vi "数据保存表格-1.vi"(1 "路径":path=path "F:/data", 2 "时间格式字符串(%c)":string="%y年%m月%d日%H 时%M 分%S秒") -> (0 "添加的路径":path)   [LabVIEW 2018]
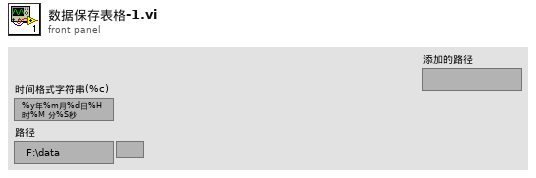
[diagram p1: front panel]
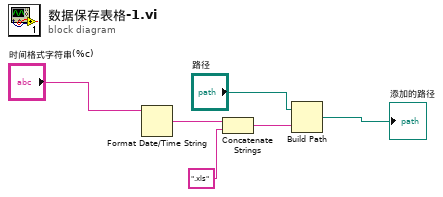
[diagram p0: block diagram]
diagram:
  n1 = Format Date/Time String(time format string (%c)="时间格式字符串(%c)") -> (date/time string=w5:string)  [unwired: 2 in]
  n2 = Concatenate Strings(w5, ".xls" ("字符串")) -> (w3:string)
  n3 = Build Path(base path="路径", name or relative path=w3) -> (appended path=→"添加的路径":path)
